vi "GIT-Current Local Branches.vi"(8 "error in":errorcluster, 11 "git-api in":refnum<class "GIT-api.lvclass">) -> (0 "error out":errorcluster, 2 "branches":string[](array[string]), 3 "git-api out":refnum<class "GIT-api.lvclass">)   [LabVIEW 2017]
doc: "show the current branch name\n\nNote: Set the \"Working Dir\" through the Git-API accessor (property node) to tell git where - in which directory - to execute this command.\n\n____\nHAMPEL SOFTWARE ENGINEERING v2.0.2 (2022-02-01 15:19)"
uses:
  <vilib>/Hampel Software Engineering/Git API/Git API/GIT-api.lvclass
panel:
  out "std out":string
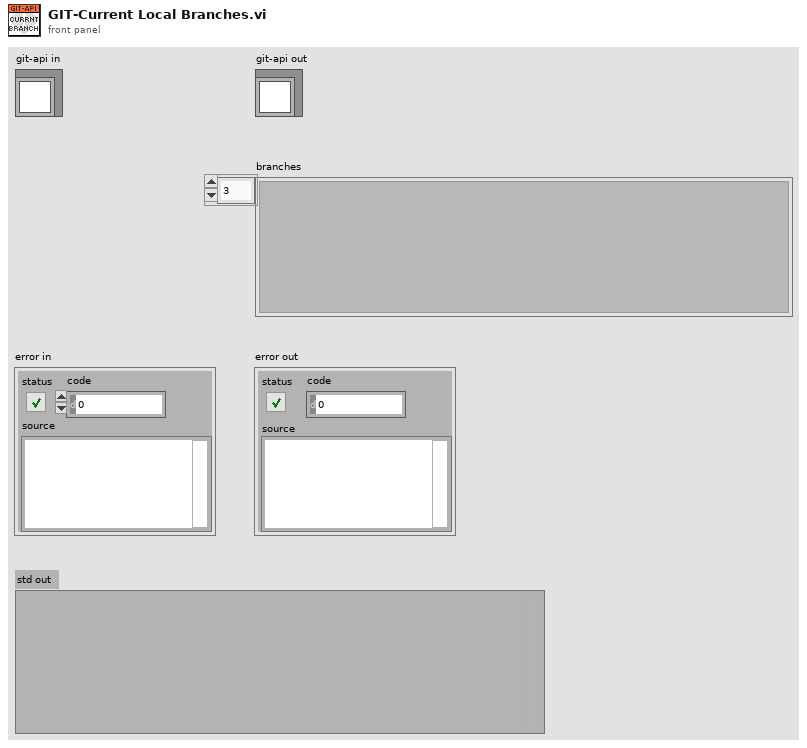
[diagram p1: front panel]
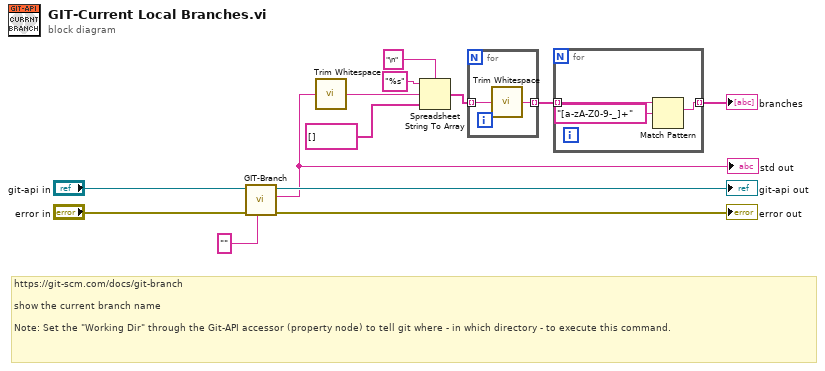
[diagram p0: block diagram]
diagram:
  # "https://git-scm.com/docs/git-branch\n\nshow the current branch name\n\nNote: Set the \"Working Dir\" through the Git-API accessor (property node) to tell git where - in which directory - to execute this command."
  n1 = call <vilib>:"GIT-Branch.vi"("param"="" ("command line"), "error in"="error in", "git-api in"="git-api in") -> ("error out"=→"error out":errorcluster, "std out"=w3:string, "git-api out"=→"git-api out":refnum<class "GIT-api.lvclass">)  [unwired: 6 in]
  "std out" <- w3
  n2 = call <vilib>:"Trim Whitespace.vi"("string"=w3) -> ("trimmed string"=w5:string)  [unwired: 1 in]
  n3 = Spreadsheet String To Array(delimiter (Tab)="\n", format string="%s", spreadsheet string=w5, array type (2D Dbl)=string[] []) -> (array=w4:string[])
  n4 = for {
    tunnel: w4 -> [w15] mode=indexing
    tunnel: [w14] -> w2 mode=indexing
    n5 = call <vilib>:"Trim Whitespace.vi"("string"=w15) -> ("trimmed string"=w14:string)  [unwired: 1 in]
  }
  n6 = for {
    tunnel: w2 -> [w18] mode=indexing
    tunnel: [w16] -> w1 mode=indexing
    n7 = Match Pattern(string=w18, regular expression="[a-zA-Z0-9-_]+") -> (match substring=w16:string)  [unwired: 1 in, 3 out]
  }
  "branches" <- w1
